vi "barra y bola labview.vi"() -> ()   [LabVIEW 2018]
uses:
  <vilib>/Instr/_visa.llb/VISA Configure Serial Port (Instr).vi
panel:
  in  "?":refnum<visa-resource-name>
  out "read buffer":string
  in  "Arduino Envio":string
  in  "Slide":dbl(slide) scale=0.0..20.0
  out "Waveform Chart":dbl(graph)
  in  "?":bool
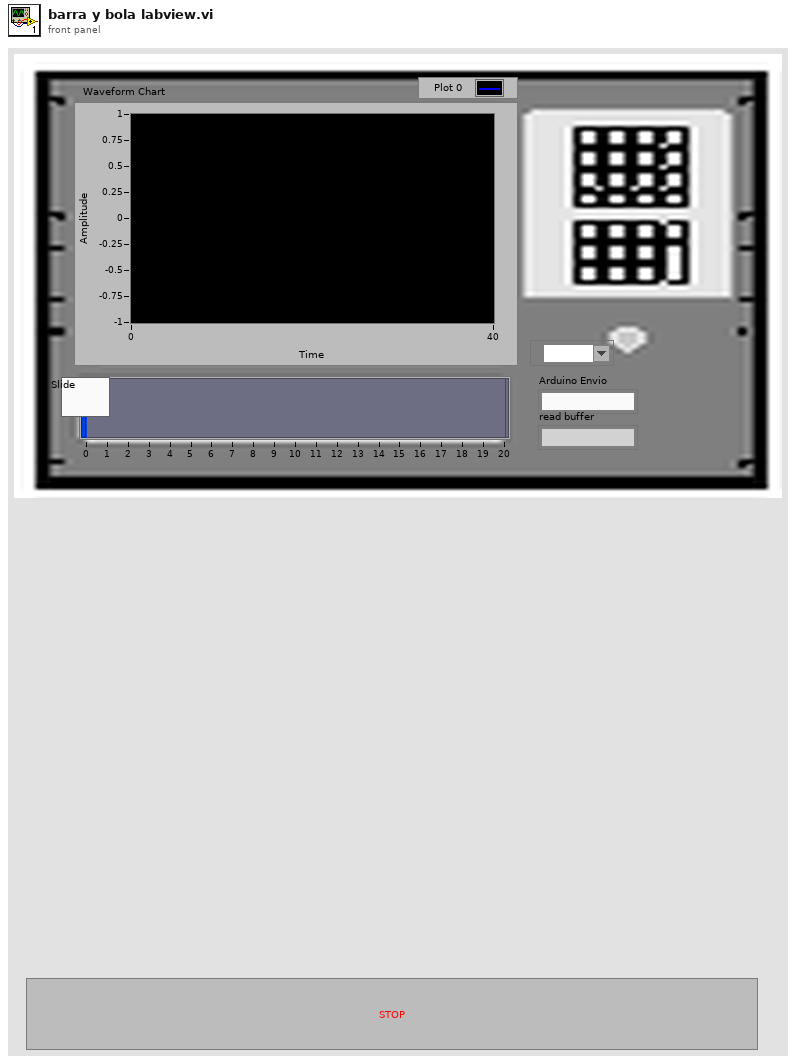
[diagram p1: front panel]
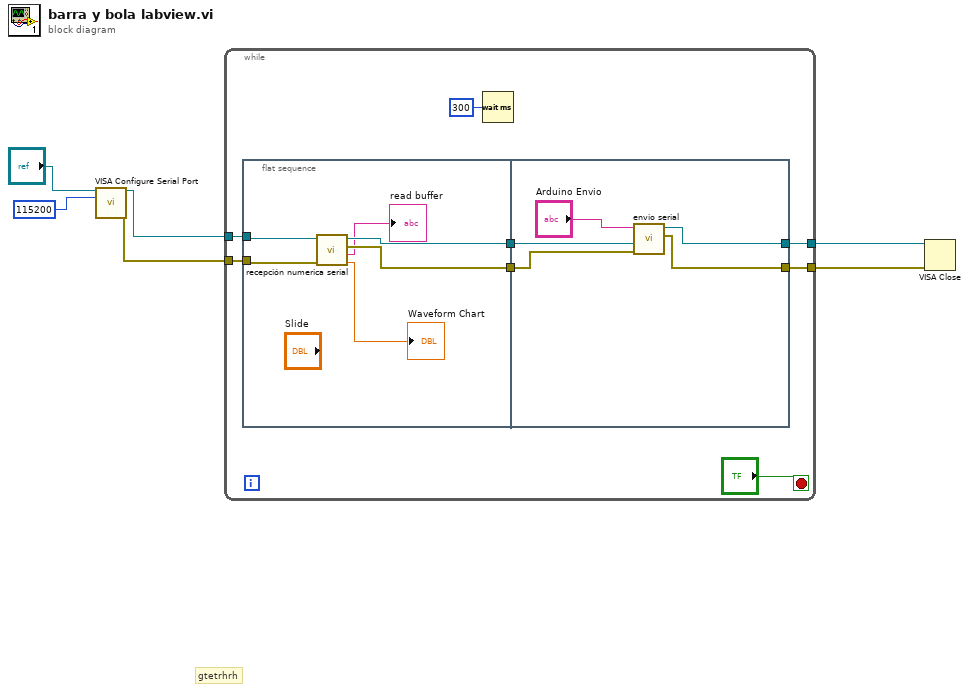
[diagram p0: block diagram]
diagram:
  # "gtetrhrh"
  n1 = call-poly "VISA Configure Serial Port"("VISA resource name"="?", "baud rate (9600)"=u32 115200) -> ("VISA resource name out"=w5:refnum<visa-resource-name>, "error out"=w3:errorcluster)  [unwired: 12 in]
  n2 = while {
    tunnel: w5 -> [w12]
    tunnel: [w10] -> w4
    tunnel: w3 -> [w9]
    tunnel: [w7] -> w2
    stop <- "?" stop-if-true
    n3 = flat-sequence {
      tunnel: w12 -> [w20]
      tunnel: [w19] -> w11
      tunnel: w9 -> [w18]
      tunnel: [w17] -> w8
      tunnel: w11 -> [w24]
      tunnel: [w25] -> w10
      tunnel: w8 -> [w22]
      tunnel: [w21] -> w7
      frame #0 {
        n4 = call "recepción numerica serial.vi"("error out"=w18, "VISA resource name out"=w20) -> ("number"=→"Waveform Chart":dbl, "read buffer"=→"read buffer":string, "error out 2"=w17:errorcluster, "VISA resource name out 2"=w19:refnum<visa-resource-name>)  [unwired: 2 in]
      }
      frame #1 {
        n5 = call "envio serial.vi"("error"=w22, "VISA resource name"=w24, "Arduino Envio"="Arduino Envio") -> ("error out"=w21:errorcluster, "VISA resource name out"=w25:refnum<visa-resource-name>)  [unwired: 3 in]
      }
    }
    n6 = Wait (ms)(milliseconds to wait=u32 300) -> ()  [unwired: 1 out]
  }
  n7 = VISA Close(VISA resource name=w4, error in (no error)=w2) -> ()  [unwired: 1 out]
